vi "Normalize_Swerve_Angles.vi"(1 "input angle [0, 360]":dbl) -> (0 "output angle [-180, 180]":dbl)   [LabVIEW 2020]
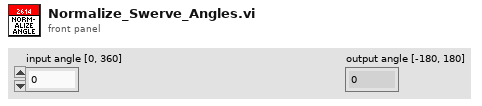
[diagram p1: front panel]
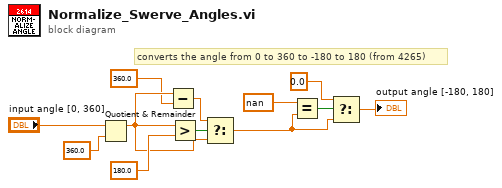
[diagram p0: block diagram]
diagram:
  # "converts the angle from 0 to 360 to -180 to 180 (from 4265)"
  n1 = Quotient & Remainder(x="input angle [0, 360]", y=360.0) -> (x-y*floor(x/y)=w5:dbl)  [unwired: 1 out]
  n2 = Subtract(x=w5, y=360.0) -> (x-y=w4:dbl)
  n3 = Greater?(x=w5, y=180.0) -> (0:w6:bool)
  n4 = Select(t=w4, s=w6, f=w5) -> (s? t:f=w11:dbl)
  n5 = Equal?(x=nan, y=w11) -> (x = y?=w10:bool)
  n6 = Select(t=0.0, s=w10, f=w11) -> (s? t:f=→"output angle [-180, 180]":dbl)
